vi "Read Gate View Trace.vi"(0 "VISA resource name":refnum<visa-resource-name>, 5 "Data (0:Positive)":i32(ring) items=["Positive", "Negative"], 7 "Start (0)":i32 min=0 max=10000, 9 "Length (1001)":i32=1001 min=1 max=10001, 11 "error in (no error)":errorcluster) -> (4 "VISA resource name out":refnum<visa-resource-name>, 6 "Gate View Trace Output":dbl[](array[numeric]), 15 "error out":errorcluster)   [LabVIEW 2020, in "Anritsu Signal Analyzer Series.lvlib"]
doc: "Reads Gate negative detection trace data when the detection mode is Positive & Negative (Normal mode)."
uses:
  Anritsu Signal Analyzer Series.lvlib
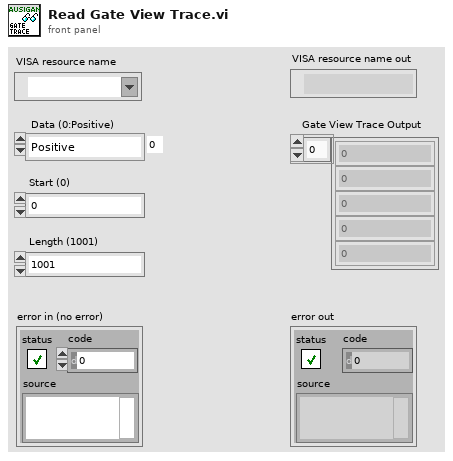
[diagram p1: front panel]
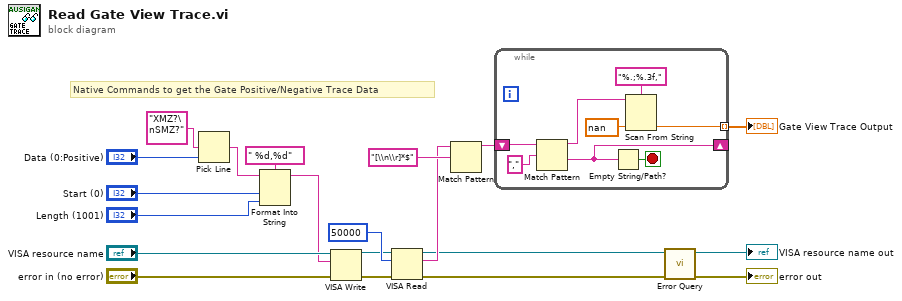
[diagram p0: block diagram]
diagram:
  # "Native Commands to get the Gate Positive/Negative Trace Data"
  n1 = Pick Line(multi-line string="XMZ?\nSMZ?" ("形式文字列"), line index="Data (0:Positive)") -> (output string=w2:string)  [unwired: 1 in]
  n2 = Format Into String(format string=" %d,%d" ("形式文字列"), initial string=w2, "Start (0)", "Length (1001)") -> (resulting string=w5:string)  [unwired: 1 in, 1 out]
  n3 = VISA Write(VISA resource name="VISA resource name", write buffer=w5, error in (no error)="error in (no error)") -> (VISA resource name out=w11:refnum<visa-resource-name>, error out=w12:errorcluster)  [unwired: 1 out]
  n4 = VISA Read(VISA resource name=w11, byte count=u32 50000 ("byte count (0)"), error in (no error)=w12) -> (VISA resource name out=w7:refnum<visa-resource-name>, read buffer=w8:string, error out=w6:errorcluster)  [unwired: 1 out]
  n5 = Match Pattern(string=w8, regular expression="[\\n\\r]*$") -> (before substring=w10:string)  [unwired: 1 in, 3 out]
  n6 = while {
    shift-right: [w21] -> _
    shift-left: w10 -> [w23]
    tunnel: [w27] -> w15 mode=indexing
    stop <- w26 stop-if-true
    n7 = Match Pattern(string=w23, regular expression=",") -> (before substring=w22:string, after substring=w21:string)  [unwired: 1 in, 2 out]
    n8 = Empty String/Path?(string/path=w21) -> (empty?=w26:bool)
    n9 = Scan From String(format string="%.;%.3f," ("Format String"), input string=w22, default 1=nan ("default value 1")) -> (output 1=w27:dbl)  [unwired: 2 in, 3 out]
  }
  "Gate View Trace Output" <- w15
  n10 = call "Error Query.vi"("error in (no error)"=w6, "VISA resource name"=w7) -> ("error out"=→"error out":errorcluster, "VISA resource name out"=→"VISA resource name out":refnum<visa-resource-name>)  [unwired: 6 in, 2 out]
